vi "Log Entry.vi"(7 "error? (F)":bool, 8 "error in (no error)":errorcluster, 9 "line text":string, 10 "line tag":string, 11 "Logging Thread in":refnum<class "Logging Thread.lvclass">) -> (0 "error out":errorcluster, 3 "Logging Thread out":refnum<class "Logging Thread.lvclass">)   [LabVIEW 2019, in "DSF Core.lvlib" / "Logging Thread.lvclass"]
uses:
  Logging Thread.lvclass
  Logging Thread.lvclass/Logging Thread.ctl
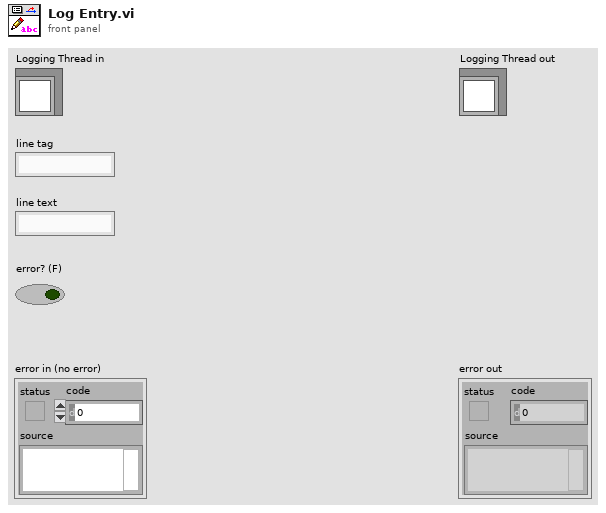
[diagram p1: front panel]
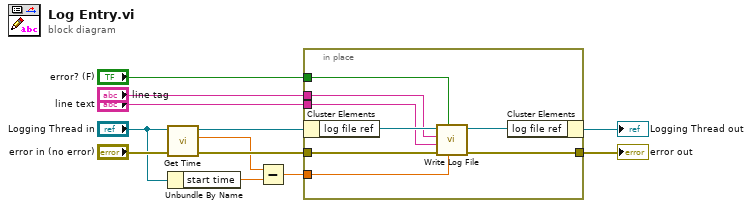
[diagram p0: block diagram]
diagram:
  n1 = call "Get Time.vi"("error in (no error)"="error in (no error)", "Logging Thread in"="Logging Thread in") -> ("error out"=w8:errorcluster, "time"=w6:dbl, "Logging Thread out"=w7:refnum<class "Logging Thread.lvclass">)  [unwired: 7 in]
  n2 = Unbundle By Name("Logging Thread in") -> ("start time"=w5:dbl)
  n3 = Subtract(x=w6, y=w5) -> (x-y=w3:dbl)
  n4 = in-place {
    in-place-border: w8 -> [w18]
    in-place-border: [w17] -> w12
    in-place-border: "line text" -> [w16]
    in-place-border: "line tag" -> [w15]
    in-place-border: w3 -> [w14]
    in-place-border: "error? (F)" -> [w13]
    n5 = in-place-cluster #1(w7) -> ("log file ref"=w20:refnum<file>)
    n6 = call "Write Log File.vi"("time"=w14, "error? (F)"=w13, "error in (no error)"=w18, "line text"=w16, "line tag"=w15, "file refnum in"=w20) -> ("error out"=w17:errorcluster, "file refnum out"=w19:refnum<file>)  [unwired: 4 in]
    n7 = in-place-cluster #1("log file ref"=w19) -> (→"Logging Thread out":refnum<class "Logging Thread.lvclass">)
  }
  "error out" <- w12
